vi "VDH-saveData.vi"(8 "error in (no error)":errorcluster, 10 "Data":T1, 11 "VDH-VNA_data_handler in":refnum<class "VDH-VNA_data_handler.lvclass">) -> (0 "error out":errorcluster, 3 "VDH-VNA_data_handler out":refnum<class "VDH-VNA_data_handler.lvclass">)   [LabVIEW 2020, in "VDH-VNA_data_handler.lvlib" / "VDH-VNA_data_handler.lvclass"]
uses:
  VDH-VNA_data_handler.lvclass
  VDH-VNA_data.ctl
  VDH-VNA_data_handler.lvclass/VDH-VNA_data_handler.ctl
  VDHI-VNA_data_handler_interface Messages/VHDI-savingStatus Msg/VHDI-savingStatus Msg.lvclass/VHDI-savingStatus Msg.ctl
  <vilib>/ActorFramework/Message Enqueuer/Message Enqueuer.lvclass/Message Enqueuer.ctl
  <vilib>/ActorFramework/Message Enqueuer/Enqueue.vi
  VDHI-VNA_data_handler_interface Messages/VHDI-savingStatus Msg/VHDI-savingStatus Msg.lvclass
  C:/Program Files (x86)/National Instruments/LabVIEW 2020/vi.lib/ActorFramework/Message/Message.lvclass
  <vilib>/ActorFramework/Message Priority Queue/Priority Enqueue.vi
  <userlib>/_OpenG.lib/file/file.llb/openg_file.lvlib
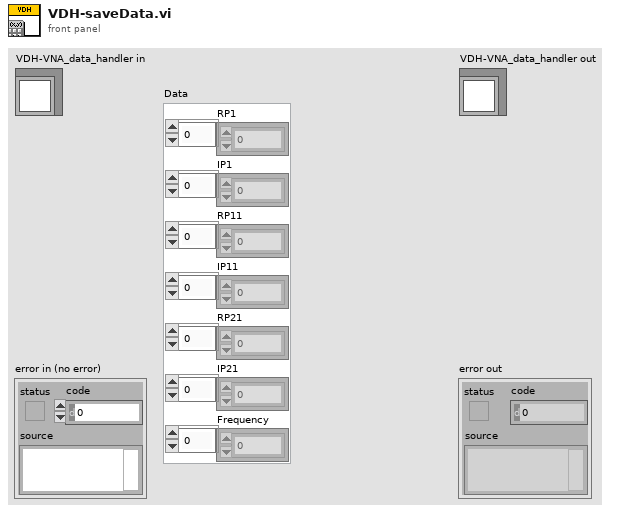
[diagram p1: front panel]
types:
  T1 = typedef "VDH-VNA_data_handler.lvlib/VDH-VNA_data_handler.lvclass/VDH-VNA_data.ctl" = cluster{"RP1":dbl[], "IP1":dbl[], "RP11":dbl[], "IP11":dbl[], "RP21":dbl[], "IP21":dbl[], "Frequency":u64[]}
  T2 = typedef "VDH-VNA_data_handler.lvlib/VDH-VNA_data_handler.lvclass/VDH-data_saving_info.ctl" = cluster{"data points left":u8, "Saving?":bool, "Folder Path":path, "filename":string}
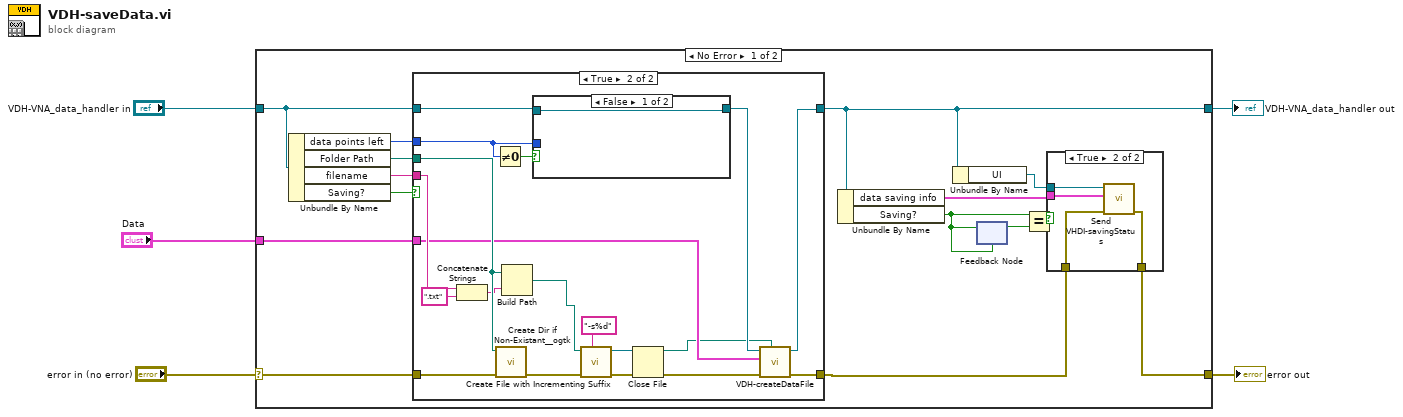
[diagram p0: block diagram]
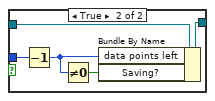
[diagram p4: hidden frame]
diagram:
  n1 = case shown="No Error" "error in (no error)" {
    selector: "error in (no error)" -> [w18 w54]
    tunnel: [w8 w54] -> w4
    tunnel: [w12 w53] -> w2
    tunnel: "VDH-VNA_data_handler in" -> [w20 w53]
    tunnel: "Data" -> [w15 _]
    frame No Error {
      n2 = Unbundle By Name(w20) -> ("data points left"=w19:u8, "Folder Path"=w17:path, "filename"=w16:string, "Saving?"=w14:bool)
      n3 = case shown="True" w14 {
        tunnel: w20 -> [w27 w46]
        tunnel: [w27 w36] -> w12
        tunnel: w19 -> [_ w45]
        tunnel: w18 -> [w26 w43]
        tunnel: [w26 w38] -> w9
        tunnel: w17 -> [_ w41]
        tunnel: w16 -> [_ w40]
        tunnel: w15 -> [_ w35]
        frame False {
        }
        frame True {
          n4 = Concatenate Strings(w40, ".txt" ("string")) -> (w29:string)
          n5 = Not Equal To 0?(x=w45) -> (x != 0?=w44:bool)
          n6 = call <userlib>:"Create Dir if Non-Existant__ogtk.vi"("error in (no error)"=w43, "Directory Path"=w41) -> ("error out"=w39:errorcluster)  [unwired: 7 in, 2 out]
          n7 = Build Path(base path=w41, name or relative path=w29) -> (appended path=w30:path)
          n8 = case shown="False" w44 {
            tunnel: w46 -> [w47 w52]
            tunnel: [w47 w51] -> w37
            tunnel: w45 -> [_ w50]
            frame False {
            }
            frame True {
              n9 = Decrement(x=w50) -> (x-1=w49:u8)
              n10 = Not Equal To 0?(x=w49) -> (x != 0?=w48:bool)
              n11 = Bundle By Name(cluster=w52, "data points left"=w49, "Saving?"=w48) -> (w51:refnum<class "VDH-VNA_data_handler.lvclass">)
            }
          }
          n12 = call <vilib>:"Create File with Incrementing Suffix.vi"("format string (\" (%d)\")"="-s%d" ("format string (\" (%d)\")"), "error in (no error)"=w39, "file path"=w30) -> ("error out"=w34:errorcluster, "refnum out"=w33:refnum<file>)  [unwired: 6 in, 1 out]
          n13 = Close File(refnum=w33, error in=w34) -> (path=w32:path, error out=w31:errorcluster)
          n14 = call "VDH-createDataFile.vi"("file path (use dialog)"=w32, "error in (no error)"=w31, "Data"=w35, "VDH-VNA_data_handler in"=w37) -> ("error out"=w38:errorcluster, "VDH-VNA_data_handler out"=w36:refnum<class "VDH-VNA_data_handler.lvclass">)  [unwired: 6 in]
        }
      }
      n15 = Unbundle By Name(w12) -> ("data saving info"=w10:T2, "Saving?"=w6:bool)
      n16 = Unbundle By Name(w12) -> ("UI"=w11:refnum<class "Message Enqueuer.lvclass">)
      n17 = feedback-in #1(w6) -> ()
      n18 = feedback #1(w6) -> (w13:bool)
      n19 = Equal?(x=w6, y=w13) -> (x = y?=w7:bool)
      n20 = case shown="True" w7 {
        tunnel: w11 -> [_ w25]
        tunnel: w10 -> [_ w24]
        tunnel: w9 -> [w21 w23]
        tunnel: [w21 w22] -> w8
        frame False {
        }
        frame True {
          n21 = call "Send VHDI-savingStatus.vi"("error in (no error)"=w23, "data saving info"=w24, "Message Enqueuer"=w25) -> ("error out"=w22:errorcluster)  [unwired: 7 in, 1 out]
        }
      }
    }
    frame Error {
    }
  }
  "error out" <- w4
  "VDH-VNA_data_handler out" <- w2
